vi "GUI_10TW_DAQmultiplier.vi"() -> ()   [LabVIEW 2013]
uses:
  shared programs/GUI_Template/GUI_master/tcp_new_data_event.ctl
  shared programs/GUI_Template/GUI_master/tcp new data cluster.ctl
panel:
  out "Backing Pressure":dbl
  out "my stuff":string[](array[string])
  out "AI_mean.Channel 7::1":dbl caption="Magnet Current Voltage - Ch7" min=0.0 max=0.0
  out "AI_mean.Channel 3::1":dbl caption="Godz Spot Z Voltage - Ch3" min=0.0 max=0.0
  out "AI_mean.Channel 2::1":dbl caption="Gas Jet Z Voltage - Ch2" min=0.0 max=0.0
  out "AI_mean.Channel 1::1":dbl caption="Gas Jet Y Voltage - Ch1" min=0.0 max=0.0
  out "AI_mean.Channel 0::1":dbl caption="Gas Jet X Voltage - Ch0" min=0.0 max=0.0
  in  "stop":bool
  out "tcp data event":T1
  out "error IO 2":errorcluster
  in  "GUIdevice 1":string="10TW_DAQ"
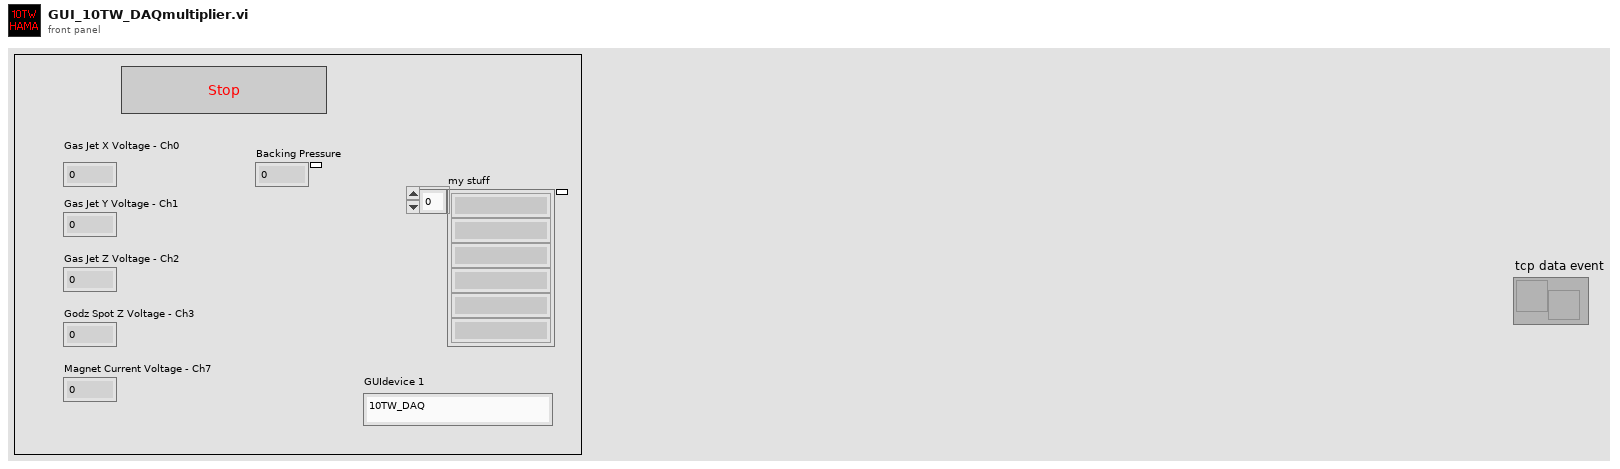
[diagram p1: front panel]
types:
  T1 = typedef "tcp_new_data_event.ctl" = refnum<user-event>
  T2 = typedef "tcp new data cluster.ctl" = cluster{"EventEnum":enum16{"new data", "connection status update"}, "Device name":string}
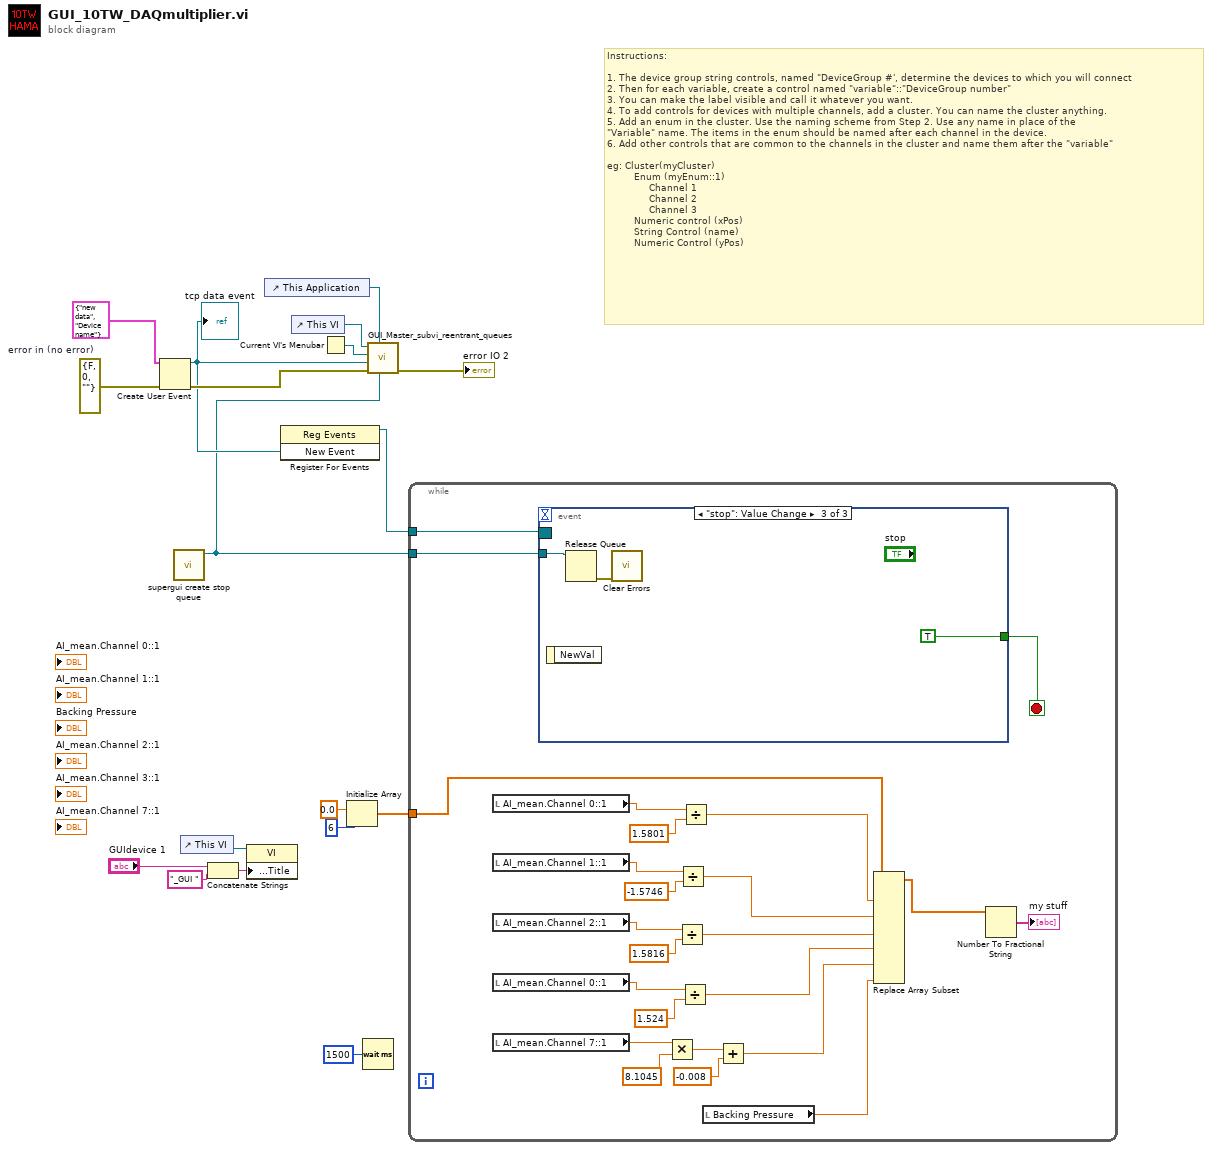
[diagram p0: block diagram]
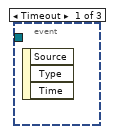
[diagram p2: hidden frame]
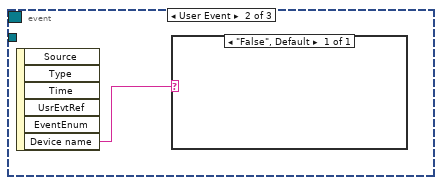
[diagram p3: hidden frame]
diagram:
  w12 = errorcluster {"status"=FALSE, "code"=0, "source"=""}  # error in (no error)
  # "Instructions:\n\n1. The device group string controls, named \"DeviceGroup #', determine the devices to which you will connect\n2. Then for each variable, create a control named \"variable\"::\"DeviceGroup number\"\n3. You can make the label visible and call it whatever you want.\n4. To add controls for devices with multiple channels, add a cluster. You can name the cluster anything.\n5. Add an enum in the cluster. Use the naming scheme from Step 2. Use any name in place of the \n\"Variable\" name. The items in the enum should be named after each channel in the device. \n6. Add other controls that are common to the channels in the cluster and name them after the \"variable\"\n\neg: Cluster(myCluster)\n         Enum (myEnum::1)\n              Channel 1 \n              Channel 2\n              Channel 3\n         Numeric control (xPos)\n         String Control (name)\n         Numeric Control (yPos)"
  n1 = Create User Event(user event datatype=T2 {"EventEnum"=enum."new data", "Device name"="Device name"} ("New Event"), error in=w12) -> (user event=w11:refnum<user-event>, error out=w14:errorcluster)
  "tcp data event" <- w11
  n2 = call "supergui create stop queue.vi"() -> ("STOP Queue out"=w5:refnum<queue>)  [unwired: 11 in]
  n3 = control-ref of="This VI"() -> (w4:refnum<vi>)
  n4 = Concatenate Strings("GUIdevice 1", "_GUI ") -> (w3:string)
  n5 = property class="VI"(reference=w4, "Front Panel.Title"=w3) -> ()  [unwired: 1 in, 2 out]
  n6 = control-ref of="This Application"() -> (w13:refnum<vi>)
  n7 = register-events(w11) -> (reference out=w10:refnum<event-registration>)  [unwired: 2 in, 1 out]
  n8 = control-ref of="This VI"() -> (w17:refnum<vi>)
  n9 = Current VI's Menubar() -> (w16:refnum<k9>)
  n10 = Initialize Array(0.0 ("element"), 6 ("dimension size")) -> (w6:dbl[])
  n11 = Wait (ms)(milliseconds to wait=u32 1500) -> ()  [unwired: 1 out]
  n12 = call "GUI_Master_subvi_reentrant_queues.vi"("STOP Queue in"=w5, "This Application"=w13, "error in (no error)"=w14, "tcp data event"=w11, "Caller menu reference"=w16, "Caller VI ref"=w17) -> ("error out"=→"error IO 2":errorcluster)  [unwired: 5 in]
  n13 = while {
    tunnel: w10 -> [w42]
    tunnel: w6 -> [w28]
    tunnel: w5 -> [w19]
    stop <- w41 stop-if-true
    n14 = local read "AI_mean.Channel 0::1"() -> (w32:dbl)
    n15 = local read "AI_mean.Channel 1::1"() -> (w31:dbl)
    n16 = local read "AI_mean.Channel 2::1"() -> (w30:dbl)
    n17 = local read "AI_mean.Channel 0::1"() -> (w29:dbl)
    n18 = local read "AI_mean.Channel 7::1"() -> (w40:dbl)
    n19 = event shown="[2] \"stop\": Value Change" {
      selector: w42 -> [_ _ _]
      dyn-events: _ -> [_ _ _]
      timeout: _ -> [_ _ _]
      tunnel: [_ _ TRUE] -> w41
      tunnel: w19 -> [_ _ w45]
      event Timeout {
        n20 = event-data() -> ()  [unwired: 1 in, 3 out]
      }
      event User Event {
        n21 = event-data() -> ("Device name"=w43:string)  [unwired: 1 in, 5 out]
        n22 = case shown="\"False\", Default" w43 {
          frame "False", Default {
          }
        }
      }
      event "stop": Value Change {
        n23 = event-data() -> ()  [unwired: 1 in, 1 out]
        n24 = Release Queue(queue=w45) -> (error out=w44:errorcluster)  [unwired: 2 in, 2 out]
        n25 = call <vilib>:"Clear Errors.vi"("error in (no error)"=w44) -> ()  [unwired: 6 in, 1 out]
      }
    }
    n26 = Multiply(x=w40, y=8.1045) -> (x*y=w37:dbl)
    n27 = Divide(x=w30, y=1.5816) -> (x/y=w25:dbl)
    n28 = Divide(x=w31, y=-1.5746) -> (x/y=w26:dbl)
    n29 = Divide(x=w29, y=1.524) -> (x/y=w24:dbl)
    n30 = Divide(x=w32, y=1.5801) -> (x/y=w27:dbl)
    n31 = local read "Backing Pressure"() -> (w20:dbl)
    n32 = Add(x=w37, y=-0.008) -> (x+y=w23:dbl)
    n33 = Replace Array Subset(array=w28, new element #1=w27, new element #2=w26, new element #3=w25, new element #4=w24, new element #5=w23, new element #6=w20) -> (w22:dbl[])  [unwired: 6 in]
    n34 = Number To Fractional String(number=w22) -> (F-format string=→"my stuff":string[])  [unwired: 3 in]
  }
